vi "DCC_find_modules_in_use.vi"(8 "Error In":errorcluster, 11 "DLL Path":path) -> (0 "Error Out":errorcluster, 1 "Module Array":i16[](array[numeric]), 2 "Number of \nUsable Modules":i16, 3 "DLL Path":path, 4 "Array of\nUsable Modules":T1[](array[typedef]), 5 "Module S/Ns":string[](array[string]))   [LabVIEW 2019]
doc: "The \"DCC_find_modules_in_use.vi\" checks which measurement card is currently in use. These which are not in use will be displayed in the \"Array Of Usable Modules\"\n\nAugust 2018\nFrank Quadt & Stefan Smietana\ninfo@becker-hickl.com"
uses:
  DCC_Controls/DCC_ModuleInfoCluster.ctl
panel:
  # "(c) 2018 Becker & Hickl GmbH\n     All Rights Reserved."
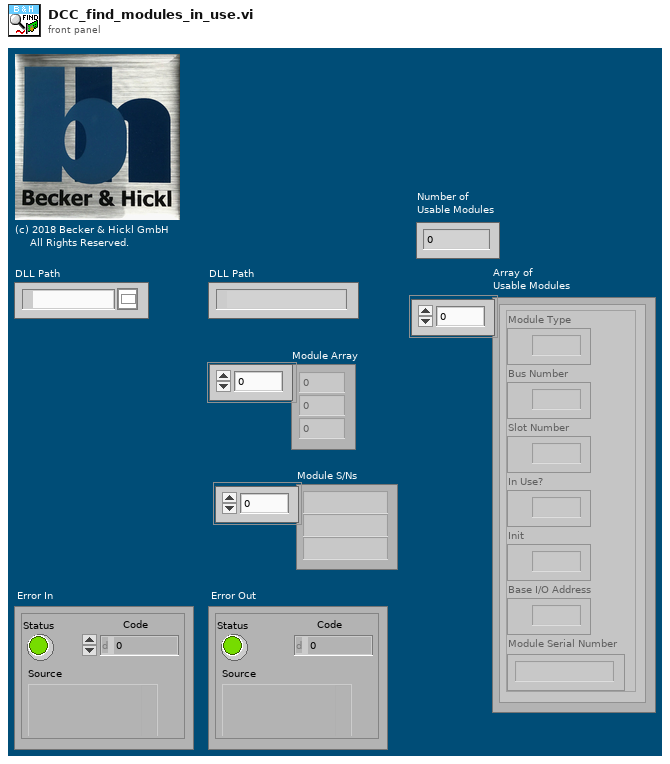
[diagram p1: front panel]
types:
  T1 = typedef "DCC_ModuleInfoCluster.ctl" = cluster{"Module Type":i16, "Bus Number":i16, "Slot Number":i16, "In Use?":i16, "Init":i16, "Base I/O Address":u16, "Module Serial Number":string}
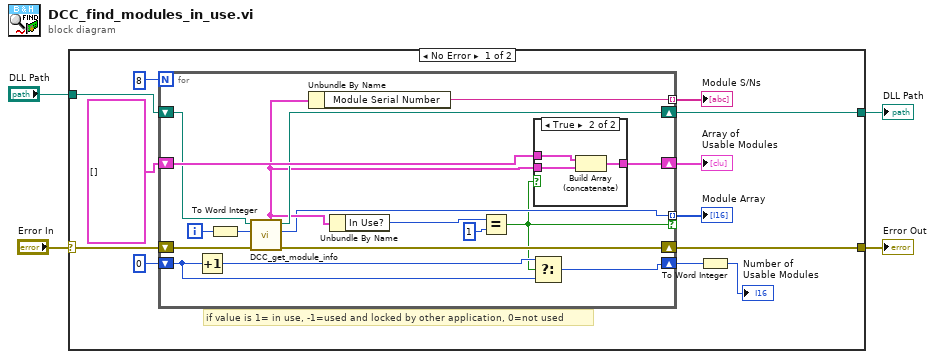
[diagram p0: block diagram]
diagram:
  n1 = case shown="No Error" "Error In" {
    selector: "Error In" -> [w11 w39]
    tunnel: [w10 w39] -> w3
    tunnel: "DLL Path" -> [w16 w38]
    tunnel: [w15 w38] -> w1
    frame No Error {
      # "if value is 1= in use, -1=used and locked by other application, 0=not used"
      n2 = for {
        N: 8 -> [_]
        shift-right: [w33] -> w12
        shift-left: T1[] [] -> [w32]
        shift-right: [w28] -> w15
        shift-left: w16 -> [w29]
        shift-right: [w26] -> w10
        shift-left: w11 -> [w27]
        shift-right: [w21] -> w8
        shift-left: 0 -> [w23]
        tunnel: [w19] -> w7 mode=indexing
        tunnel: [w18] -> w5 mode=indexing if=w17
        i -> [w25]
        n3 = Increment(x=w23) -> (x+1=w22:i32)
        n4 = To Word Integer(number=w25) -> (16bit integer=w24:i16)
        n5 = call "DCC_get_module_info.vi"("Error In"=w27, "Module No"=w24, "DLL Path"=w29) -> ("Error Out"=w26:errorcluster, "Module No"=w18:i16, "DLL Path"=w28:path, "Module Info"=w20:T1)  [unwired: 5 in]
        n6 = Unbundle By Name(w20) -> ("Module Serial Number"=w19:string)
        n7 = Unbundle By Name(w20) -> ("In Use?"=w31:i16)
        n8 = Equal?(x=w31, y=i16 1) -> (x = y?=w17:bool)
        n9 = Select(t=w22, s=w17, f=w23) -> (s? t:f=w21:i32)
        n10 = case shown="True" w17 {
          tunnel: w20 -> [_ w37]
          tunnel: [w34 w36] -> w33
          tunnel: w32 -> [w34 w35]
          frame False {
          }
          frame True {
            n11 = Build Array (concatenate)(w35, w37) -> (w36:T1[])
          }
        }
      }
      "Array of\nUsable Modules" <- w12
      "Module Array" <- w5
      "Module S/Ns" <- w7
      n12 = To Word Integer(number=w8) -> (16bit integer=→"Number of \nUsable Modules":i16)
    }
    frame Error {
    }
  }
  "Error Out" <- w3
  "DLL Path" <- w1
